vi "Destroy.vi"(0 "scripts manager in":refnum<class "scripts manager.lvclass">, 11 "error in (no error)":errorcluster) -> (4 "scripts manager out":refnum<class "scripts manager.lvclass">, 15 "error out":errorcluster)   [LabVIEW 2019, in "LSL.lvlib" / "scripts manager.lvclass"]
uses:
  scripts manager.lvclass
  functions/functionsbase/functionbase.lvclass
  common/line and indent/Line Details.ctl
  output terminal/Base/Output Terminal.lvclass
  variables/RT Variables/RT Variables.lvclass
  scripts manager.lvclass/scripts manager.ctl
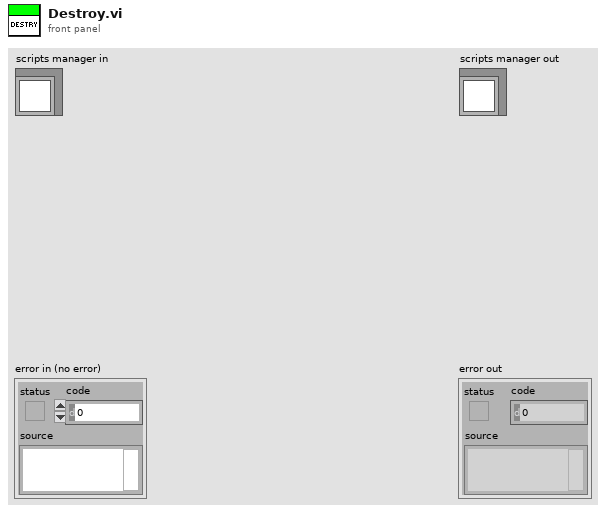
[diagram p1: front panel]
types:
  T1 = typedef "Line Details.ctl" = cluster{"Line#":i64, "Indent#":i64, "Function":string}
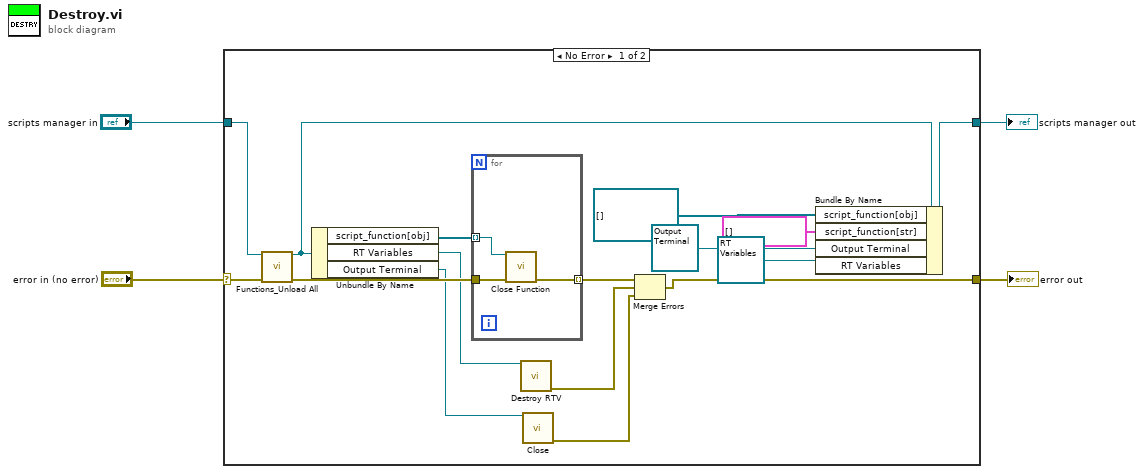
[diagram p0: block diagram]
diagram:
  n1 = case shown="No Error" "error in (no error)" {
    selector: "error in (no error)" -> [w20 w25]
    tunnel: [w15 w25] -> w3
    tunnel: [w13 w24] -> w1
    tunnel: "scripts manager in" -> [w19 w24]
    frame No Error {
      n2 = call-dynamic "Functions_Unload All.vi"("scripts manager in"=w19, "error in (no error)"=w20) -> ("scripts manager out"=w14:refnum<class "scripts manager.lvclass">, "error out"=w17:errorcluster)  [unwired: 12 in]
      n3 = Unbundle By Name(w14) -> ("script_function[obj]"=w18:refnum<class "functionbase.lvclass">[], "RT Variables"=w9:refnum<class "RT Variables.lvclass">, "Output Terminal"=w8:refnum<class "Output Terminal.lvclass">)
      n4 = for {
        tunnel: w18 -> [w23] mode=indexing
        tunnel: w17 -> [w22]
        tunnel: [w21] -> w16 mode=indexing
        n5 = call-dynamic "Close Function.vi"("functionbase in"=w23, "error in (no error)"=w22) -> ("error out"=w21:errorcluster)  [unwired: 12 in, 1 out]
      }
      n6 = call-dynamic "Destroy RTV.vi"("RT Variables"=w9) -> ("error out"=w10:errorcluster)  [unwired: 13 in, 1 out]
      n7 = call-dynamic "Close.vi"("Output Terminal in"=w8) -> ("error out"=w7:errorcluster)  [unwired: 13 in, 1 out]
      n8 = Merge Errors(w16, w10, w7) -> (w15:errorcluster)
      n9 = Bundle By Name(cluster=w14, "script_function[obj]"=refnum<class "functionbase.lvclass">[] [], "script_function[str]"=T1[] [], "Output Terminal"=refnum<class "Output Terminal.lvclass"> refnum, "RT Variables"=refnum<class "RT Variables.lvclass"> refnum) -> (w13:refnum<class "scripts manager.lvclass">)
    }
    frame Error {
    }
  }
  "error out" <- w3
  "scripts manager out" <- w1
